vi "Elavator_Motor_Value_Max_Speed.vi"(6 "Ele_Pos":dbl, 8 "Pos_Des":dbl, 9 "Pos_Active":bool, 11 "Ele_Manual":dbl) -> (2 "Ele_At_Pos":bool, 3 "Ele_Lift_Power":dbl)   [LabVIEW 2014]
panel:
  in  "lower limit":dbl=8.25
  in  "upper limit":dbl=53.5
  out "Pos_Power_Map":cluster{"Speed X":dbl[], "Speed Y":dbl[]}(graph)
  in  "Y_Array":dbl[](array[numeric])=[1.0, 0.15, 0.15, 0.0, -0.15, -0.15, -1.0] format="%.2f"
  in  "X_Array":dbl[](array[numeric])=[-1.0, -0.1, -0.01, 0.0, 0.01, 0.1, 1.0, 0.0, 0.0, 0.0, 100.0] format="%.2f"
  out "y_out":dbl
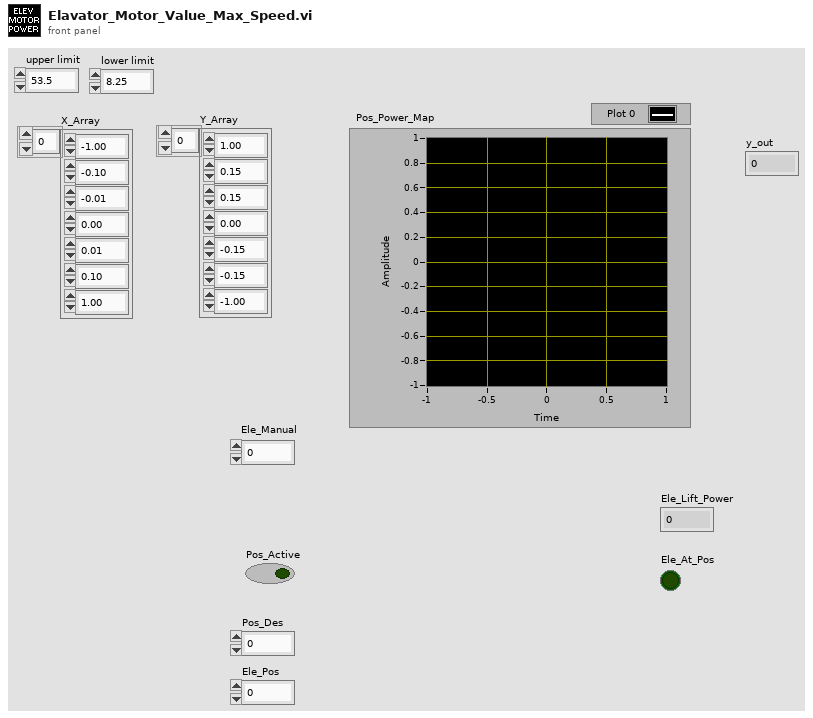
[diagram p1: front panel]
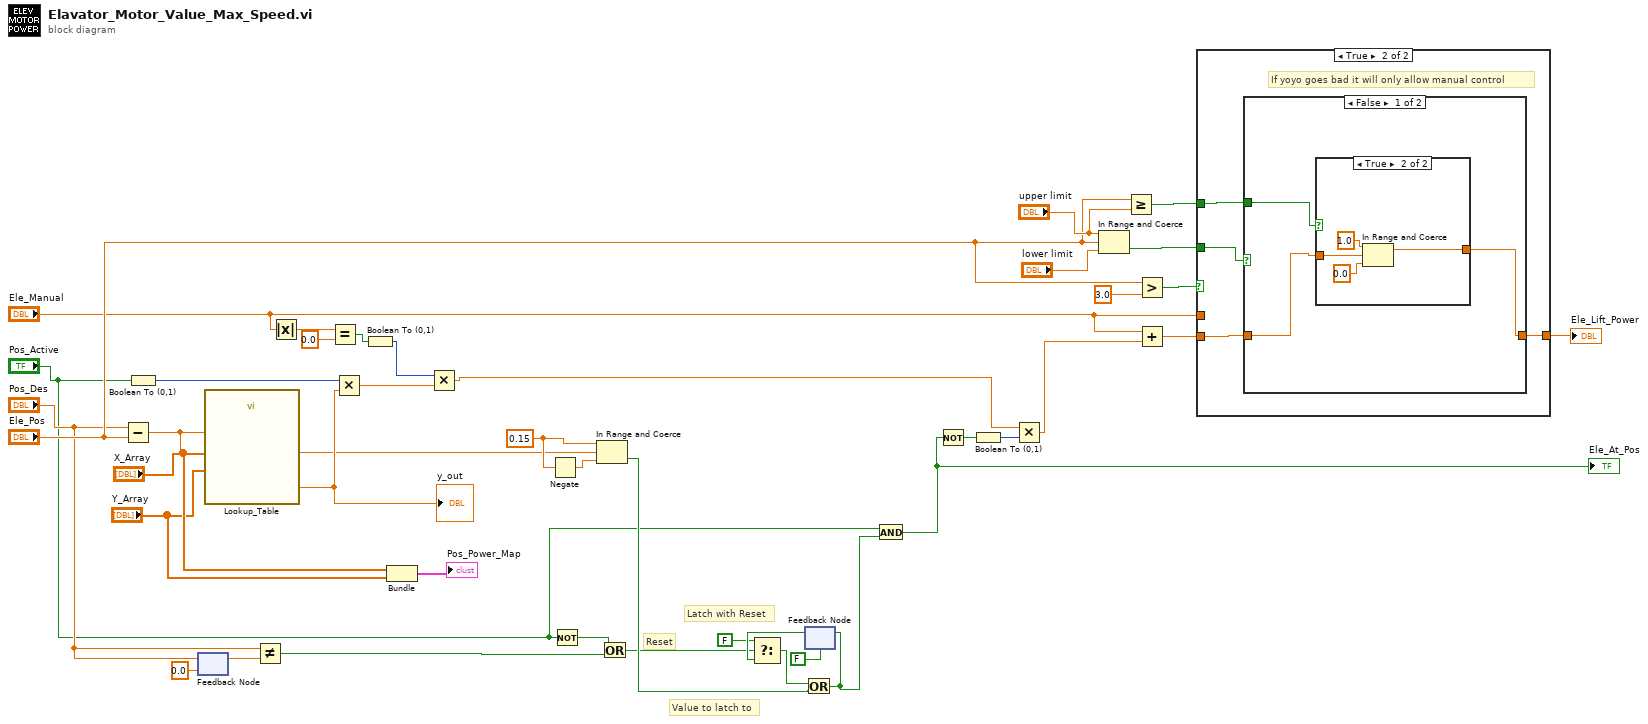
[diagram p0: block diagram]
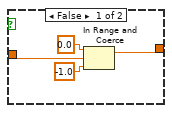
[diagram p3: hidden frame]
diagram:
  w30 = 0.15 ("upper limit")
  # "Value to latch to"
  # "Reset"
  # "Latch with Reset"
  n1 = Subtract(x="Pos_Des", y="Ele_Pos") -> (x-y=w29:dbl)
  n2 = Boolean To (0,1)(Boolean="Pos_Active") -> (0, 1=w39:i16)
  n3 = feedback #1(0.0 ("Pos_Des")) -> (w16:dbl)
  n4 = feedback-in #1("Pos_Des") -> ()
  n5 = call "Lookup_Table.vi"("Y_Array"="Y_Array", "x_in"=w29, "X_Array"="X_Array") -> ("y_out"=w35:dbl)  [unwired: 6 in]
  "y_out" <- w35
  n6 = Not Equal?(x="Pos_Des", y=w16) -> (x != y?=w9:bool)
  n7 = Absolute Value(x="Ele_Manual") -> (abs(x)=w40:dbl)
  n8 = Equal?(x=w40, y=0.0) -> (x = y?=w38:bool)
  n9 = Multiply(x=w39, y=w35) -> (x*y=w36:dbl)
  n10 = Boolean To (0,1)(Boolean=w38) -> (0, 1=w37:i16)
  n11 = Bundle("X_Array"="X_Array", "Y_Array"="Y_Array") -> (→"Pos_Power_Map":cluster{"X_Array":dbl[], "Y_Array":dbl[]})  [unwired: 1 in]
  n12 = Multiply(x=w37, y=w36) -> (x*y=w2:dbl)
  n13 = Negate(x=w30) -> (-x=w31:dbl)
  n14 = Not(x="Pos_Active") -> (.not. x?=w7:bool)
  n15 = In Range and Coerce(upper limit=w30, x=w29, lower limit=w31) -> (In Range?=w10:bool)  [unwired: 1 out]
  n16 = Or(x=w7, y=w9) -> (x .or. y?=w8:bool)
  n17 = feedback #2(FALSE) -> (w12:bool)
  n18 = Select(t=FALSE, s=w8, f=w12) -> (s? t:f=w13:bool)
  n19 = Or(x=w13, y=w10) -> (x .or. y?=w6:bool)
  n20 = feedback-in #2(w6) -> ()
  n21 = And(x="Pos_Active", y=w6) -> (x .and. y?=w5:bool)
  "Ele_At_Pos" <- w5
  n22 = Not(x=w5) -> (.not. x?=w18:bool)
  n23 = Boolean To (0,1)(Boolean=w18) -> (0, 1=w19:i16)
  n24 = Multiply(x=w2, y=w19) -> (x*y=w1:dbl)
  n25 = In Range and Coerce(upper limit="upper limit", x="Ele_Pos", lower limit="lower limit") -> (In Range?=w28:bool)  [unwired: 1 out]
  n26 = Greater Or Equal?(x="Ele_Pos", y="upper limit") -> (x >= y?=w25:bool)
  n27 = Greater?(x="Ele_Pos", y=3.0) -> (0:w23:bool)
  n28 = Add(x="Ele_Manual", y=w1) -> (x+y=w27:dbl)
  n29 = case shown="True" w23 {
    tunnel: w28 -> [_ w46]
    tunnel: w27 -> [_ w45]
    tunnel: [w42 w44] -> w3
    tunnel: w25 -> [_ w43]
    tunnel: "Ele_Manual" -> [w42 _]
    frame False {
      # "Failure mode"
    }
    frame True {
      # "If yoyo goes bad it will only allow manual control"
      n30 = case shown="False" w46 {
        tunnel: w45 -> [w48 w58]
        tunnel: [w47 w58] -> w44
        tunnel: w43 -> [w49 _]
        frame False {
          n31 = case shown="True" w49 {
            tunnel: w48 -> [w51 w57]
            tunnel: [w50 w54] -> w47
            frame False {
              n32 = In Range and Coerce(upper limit=0.0, x=w51, lower limit=-1.0) -> (coerced(x)=w50:dbl)  [unwired: 1 out]
            }
            frame True {
              n33 = In Range and Coerce(upper limit=1.0, x=w57, lower limit=0.0) -> (coerced(x)=w54:dbl)  [unwired: 1 out]
            }
          }
        }
        frame True {
        }
      }
    }
  }
  "Ele_Lift_Power" <- w3
